vi "Autonomous Independent.vi"() -> ()   [LabVIEW 2014]
doc: "This VI is called when autonomous begins, and will automatically be terminated when autonomous ends. You can carry out timed or sensor driven robot movement independently without needing to return to the caller."
uses:
  <vilib>/Rock Robotics/WPI/Joystick/WPI_JoystickGetSetRefNum.vi
  Robot Global Data.vi
  <vilib>/Rock Robotics/WPI/RobotDrive/WPI_RobotDriveArcadeDrive_Standard(NoSaturation).vi
  <vilib>/Rock Robotics/WPI/SafetyOutput/WPI_SafetyOutputConfigMenu.ctl
  <vilib>/Rock Robotics/WPI/Relay/WPI_RelayValue.ctl
panel:
  out "Current Movement, for debugging":T1 {"Y Joystick Value" scale=1.0..-1.0; "X Joystick Value" scale=-1.0..1.0}
  in  "Array of robot movements":T2(array[cluster]) {"Y Joystick Value" scale=1.0..-1.0; "X Joystick Value" scale=-1.0..1.0}
  # "Be sure to right-click and choose Data Operations>>Make Current Value default if you want to save the array values with the VI"
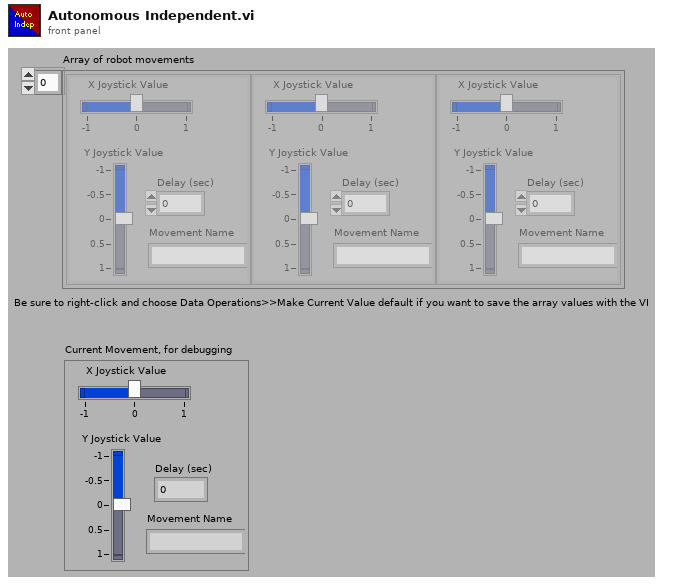
[diagram p1: front panel]
types:
  T1 = cluster{"X Joystick Value":dbl, "Y Joystick Value":dbl, "Delay (sec)":dbl, "Movement Name":string}
  T2 = cluster{"X Joystick Value":dbl, "Y Joystick Value":dbl, "Delay (sec)":dbl, "Movement Name":string}[]
  T3 = typedef "WPI_SafetyOutputConfigMenu.ctl" = enum16{"Enable", "Disable"}
  T4 = typedef "WPI_RelayValue.ctl" = enum16{"Off", "On", "Forward", "Reverse"}
  T5 = typedef "WPI_RobotDriveDevRef.ctl" = cluster{"DevStatus":errorcluster, "Motors[]":T6[], "Square Inputs":bool, "Max Output":dbl}
  T6 = typedef "WPI_MotorControlDeviceRef.ctl" = cluster{"DeviceStatus":errorcluster, "Type":enum16{"PWM", "CAN"}, "PWM":cluster{"Digital Module":T7, "PWM Channel":T8, "DeadBand":T9}, "CAN":cluster{"Device Number":u8, "Control Mode":T10, "Semaphore":T11, "Max Vout":dbl}, "Invert":bool, "TransformRef":T12, "InvTransformRef":T12}
  T7 = typedef "FPGA_TypedefDigitalModule.ctl" = enum16{"Digital Module 1", "Digital Module 2"}
  T8 = typedef "FPGA_DIOPWMChannel.ctl" = enum8{"PWM 1", "PWM 2", "PWM 3", "PWM 4", "PWM 5", "PWM 6", "PWM 7", "PWM 8", "PWM 9", "PWM 10", "Invalid"}
  T9 = typedef "WPI_PWMDeadband.ctl" = cluster{"Name":string, "maxPositivePwm":i32, "minPositivePwm":i32, "centerPwm":i32, "maxNegativePwm":i32, "minNegativePwm":i32, "angularRange":u16}
  T10 = typedef "WPI_CANJaguar_ControlMode.ctl" = enum8{"Percent VBus", "Current", "Speed", "Position", "Voltage"}
  T11 = typedef "Semaphore RefNum" = refnum<k1>
  T12 = typedef "WPI_PWMTransform_ConPane.ctl" = refnum<vi>
  T13 = typedef "WPI_GyroDevRef.ctl" = cluster{"DevStatus":errorcluster, "Analog Module":T14, "Analog Channel":T15, "Offset":dbl, "Gain (VoltsPerDegree/Second)":dbl}
  T14 = typedef "FPGA_TypedefAnalogModule.ctl" = enum16{"Analog Module 1", "Analog Module 2"}
  T15 = typedef "FPGA_AIChannel.ctl" = enum8{"AI 1", "AI 2", "AI 3", "AI 4", "AI 5", "AI 6", "AI 7", "AI 8", "Invalid"}
  T16 = typedef "WPI_RelayDevRef.ctl" = cluster{"DevStatus":errorcluster, "Relay Channel":T17, "Digital Module":T7, "Relay Direction":T18}
  T17 = typedef "FPGA_DIORelayChannel.ctl" = enum8{"Relay 1", "Relay 2", "Relay 3", "Relay 4", "Relay 5", "Relay 6", "Relay 7", "Relay 8", "Invalid"}
  T18 = typedef "WPI_RelayDirection.ctl" = enum16{"Both directions", "Forward only", "Reverse only"}
  T19 = typedef "WPI_JoystickDevRef.ctl" = cluster{"Device":T20}
  T20 = typedef "WPI_JoystickDeviceEnum.ctl" = enum16{"USB 0", "USB 1", "USB 2", "USB 3", "USB 4", "USB 5"}
  T21 = cluster{"axis 1 (x)":dbl, "axis 2 (y)":dbl, "axis 3 (throttle)":dbl, "axis 4":dbl, "axis 5":dbl, "axis 6":dbl}
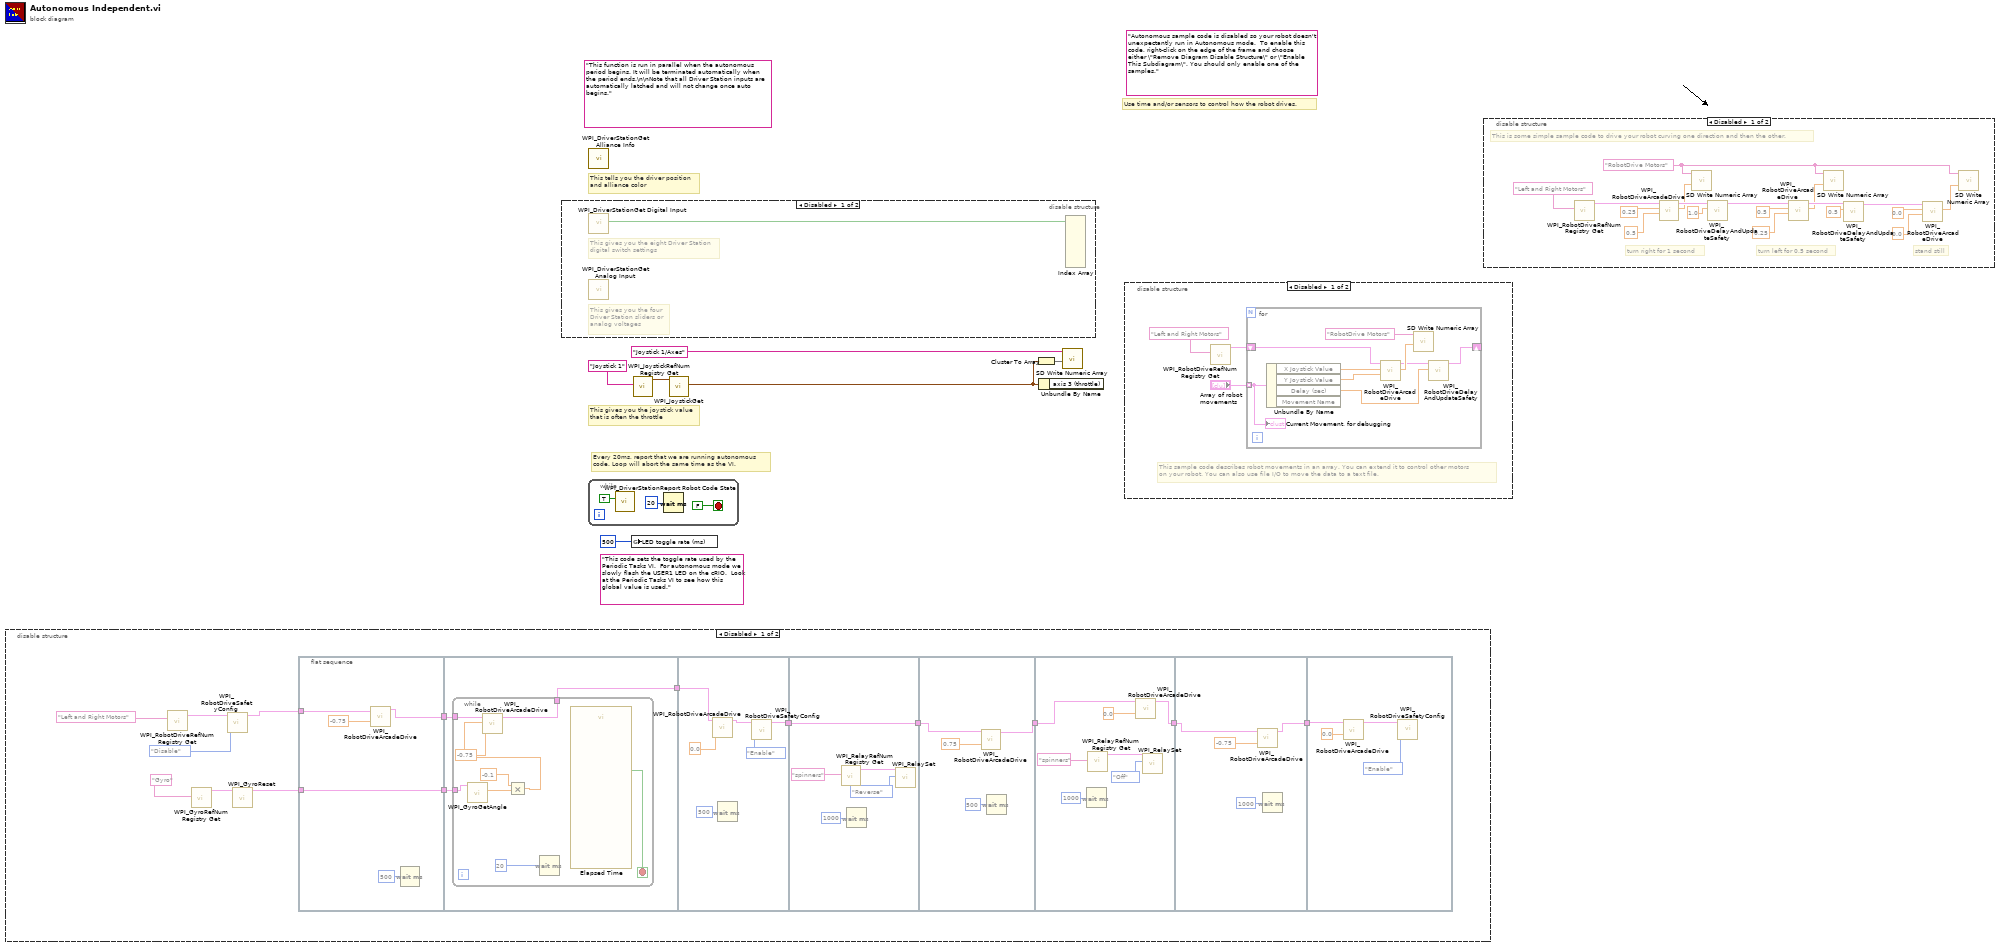
[diagram p0: block diagram]
diagram:
  (unwired) "This code sets the toggle rate used by the Periodic Tasks VI.  For autonomous mode we slowly flash the USER1 LED on the cRIO.  Look at the Periodic Tasks VI to see how this global value is used."
  (unwired) "Autonomous sample code is disabled so your robot doesn't unexpectantly run in Autonomous mode.  To enable this code, right-click on the edge of the frame and choose either \"Remove Diagram Disable Structure\" or \"Enable This Subdiagram\". You should only enable one of the samples."
  (unwired) "This function is run in parallel when the autonomous period begins. It will be terminated automatically when the period ends.\n\nNote that all Driver Station inputs are automatically latched and will not change once auto begins."
  # "Every 20ms, report that we are running autonomous\ncode. Loop will abort the same time as the VI."
  # "This gives you the joystick value\nthat is often the throttle"
  # "Use time and/or sensors to control how the robot drives."
  # "This tells you the driver position\nand alliance color"
  n1 = disable-structure shown="Disabled" {
    frame Disabled {
      n2 = call <vilib>:"WPI_RobotDriveRefNum Registry Get.vi"("refnum name"="Left and Right Motors") -> ("RobotDriveDevRef"=w12:T5)  [unwired: 9 in, 1 out]
      n3 = call <vilib>:"WPI_GyroRefNum Registry Get.vi"("refnum name"="Gyro") -> ("GyroDevRef"=w7:T13)  [unwired: 9 in, 1 out]
      n4 = call <vilib>:"WPI_RobotDriveSafetyConfig.vi"("mode"=WPI_SafetyOutputConfigMenu."Disable", "RobotDriveDevRef"=w12) -> ("RobotDriveDevRef"=w10:T5)  [unwired: 8 in, 1 out]
      n5 = call <vilib>:"WPI_GyroReset.vi"("GyroDevRef"=w7) -> ("GyroDevRef"=w9:T13)  [unwired: 9 in, 1 out]
      n6 = flat-sequence {
        tunnel: [w24] -> w21
        tunnel: w10 -> [w25]
        tunnel: w9 -> [w23]
        tunnel: [w23] -> w20
        tunnel: w21 -> [w27]
        tunnel: w20 -> [w28]
        tunnel: [w29] -> w19
        tunnel: [w40] -> w18
        tunnel: w19 -> [w41]
        tunnel: w18 -> [w49]
        tunnel: [w49] -> w17
        tunnel: w17 -> [w50]
        tunnel: [w51] -> w16
        tunnel: w16 -> [w58]
        tunnel: [w57] -> w15
        tunnel: w15 -> [w62]
        tunnel: [w61] -> w14
        tunnel: w14 -> [w65]
        frame #0 {
          n7 = call-poly <vilib>:"WPI_RobotDriveArcadeDrive.vi"("Y axis value"=-0.75, "RobotDriveDevRef"=w25) -> ("RobotDriveDevRef"=w24:T5)  [unwired: 7 in, 2 out]
          n8 = Wait (ms)(milliseconds to wait=u32 500) -> ()  [unwired: 1 out]
        }
        frame #1 {
          n9 = while {
            tunnel: [w31] -> w29
            tunnel: w28 -> [w36]
            tunnel: w27 -> [w32]
            stop <- w38 stop-if-true
            n10 = call <vilib>:"WPI_GyroGetAngle.vi"("GyroDevRef"=w36) -> ("Angle"=w34:dbl)  [unwired: 7 in, 3 out]
            n11 = Multiply(x=-0.1, y=w34) -> (x*y=w33:dbl)
            n12 = call-poly <vilib>:"WPI_RobotDriveArcadeDrive.vi"("Y axis value"=-0.75, "X axis value"=w33, "RobotDriveDevRef"=w32) -> ("RobotDriveDevRef"=w31:T5)  [unwired: 6 in, 2 out]
            n13 = Wait (ms)(milliseconds to wait=u32 20) -> ()  [unwired: 1 out]
            n14 = call "Elapsed Time"() -> ("Time has Elapsed"=w38:bool)  [unwired: 12 in, 7 out]
          }
        }
        frame #2 {
          n15 = call-poly <vilib>:"WPI_RobotDriveArcadeDrive.vi"("Y axis value"=0.0, "RobotDriveDevRef"=w41) -> ("RobotDriveDevRef"=w43:T5)  [unwired: 7 in, 2 out]
          n16 = Wait (ms)(milliseconds to wait=u32 500) -> ()  [unwired: 1 out]
          n17 = call <vilib>:"WPI_RobotDriveSafetyConfig.vi"("mode"=WPI_SafetyOutputConfigMenu."Enable", "RobotDriveDevRef"=w43) -> ("RobotDriveDevRef"=w40:T5)  [unwired: 8 in, 1 out]
        }
        frame #3 {
          n18 = call <vilib>:"WPI_RelayRefNum Registry Get.vi"("refnum name"="spinners") -> ("RelayDevRef"=w46:T16)  [unwired: 9 in, 1 out]
          n19 = Wait (ms)(milliseconds to wait=u32 1000) -> ()  [unwired: 1 out]
          n20 = call <vilib>:"WPI_RelaySet.vi"("RelayValue"=WPI_RelayValue."Reverse", "RelayDevRef"=w46) -> ()  [unwired: 8 in, 2 out]
        }
        frame #4 {
          n21 = call-poly <vilib>:"WPI_RobotDriveArcadeDrive.vi"("Y axis value"=0.75, "RobotDriveDevRef"=w50) -> ("RobotDriveDevRef"=w51:T5)  [unwired: 7 in, 2 out]
          n22 = Wait (ms)(milliseconds to wait=u32 500) -> ()  [unwired: 1 out]
        }
        frame #5 {
          n23 = Wait (ms)(milliseconds to wait=u32 1000) -> ()  [unwired: 1 out]
          n24 = call <vilib>:"WPI_RelayRefNum Registry Get.vi"("refnum name"="spinners") -> ("RelayDevRef"=w56:T16)  [unwired: 9 in, 1 out]
          n25 = call-poly <vilib>:"WPI_RobotDriveArcadeDrive.vi"("Y axis value"=0.0, "RobotDriveDevRef"=w58) -> ("RobotDriveDevRef"=w57:T5)  [unwired: 7 in, 2 out]
          n26 = call <vilib>:"WPI_RelaySet.vi"("RelayValue"=WPI_RelayValue."Off", "RelayDevRef"=w56) -> ()  [unwired: 8 in, 2 out]
        }
        frame #6 {
          n27 = call-poly <vilib>:"WPI_RobotDriveArcadeDrive.vi"("Y axis value"=-0.75, "RobotDriveDevRef"=w62) -> ("RobotDriveDevRef"=w61:T5)  [unwired: 7 in, 2 out]
          n28 = Wait (ms)(milliseconds to wait=u32 1000) -> ()  [unwired: 1 out]
        }
        frame #7 {
          n29 = call-poly <vilib>:"WPI_RobotDriveArcadeDrive.vi"("Y axis value"=0.0, "RobotDriveDevRef"=w65) -> ("RobotDriveDevRef"=w67:T5)  [unwired: 7 in, 2 out]
          n30 = call <vilib>:"WPI_RobotDriveSafetyConfig.vi"("mode"=WPI_SafetyOutputConfigMenu."Enable", "RobotDriveDevRef"=w67) -> ()  [unwired: 8 in, 2 out]
        }
      }
    }
    frame Enabled {
    }
  }
  n31 = disable-structure shown="Disabled" {
    frame Disabled {
      # "This gives you the eight Driver Station\ndigital switch settings"
      # "This gives you the four\nDriver Station sliders or\nanalog voltages"
      n32 = call <vilib>:"WPI_DriverStationGet Digital Input.vi"() -> ("Driver Station Digital Input (1-8)"=w69:bool[])  [unwired: 11 out]
      n33 = call <vilib>:"WPI_DriverStationGet Analog Input.vi"() -> ()  [unwired: 12 out]
      n34 = Index Array(array=w69) -> ()  [unwired: 8 in, 8 out]
    }
    frame Enabled {
    }
  }
  n35 = while {
    stop <- FALSE stop-if-true
    n36 = call <vilib>:"WPI_DriverStationReport Robot Code State.vi"("Autonomous"=TRUE) -> ()  [unwired: 10 in, 1 out]
    n37 = Wait (ms)(milliseconds to wait=u32 20) -> ()  [unwired: 1 out]
  }
  n38 = call <vilib>:"WPI_DriverStationGet Alliance Info.vi"() -> ()  [unwired: 12 out]
  n39 = global write "Robot Global Data.vi" "LED toggle rate (ms)"(u32 500 ("LED ms toggle rate")) -> ()
  n40 = call <vilib>:"WPI_JoystickRefNum Registry Get.vi"("refnum name"="Joystick 1") -> ("JoystickDevRef"=w5:T19)  [unwired: 1 in, 9 out]
  n41 = call <vilib>:"WPI_JoystickGet.vi"("JoystickDevRef"=w5) -> ("Axes"=w2:T21)  [unwired: 1 in, 5 out]
  n42 = Cluster To Array(cluster=w2) -> (array=w3:dbl[])
  n43 = Unbundle By Name(w2) -> ()  [unwired: 1 out]
  n44 = call <vilib>:"SD Write Numeric Array.vi"("Numeric Array"=w3, "Name"="Joystick 1/Axes") -> ()  [unwired: 8 in, 2 out]
  n45 = disable-structure shown="Disabled" {
    frame Disabled {
      # "This sample code describes robot movements in an array. You can extend it to control other motors\non your robot. You can also use file I/O to move the data to a text file."
      n46 = call <vilib>:"WPI_RobotDriveRefNum Registry Get.vi"("refnum name"="Left and Right Motors") -> ("RobotDriveDevRef"=w74:T5)  [unwired: 1 in, 9 out]
      n47 = for {
        shift-right: [w80] -> _
        shift-left: w74 -> [w81]
        tunnel: "Array of robot movements" -> [w76] mode=indexing
        n48 = Unbundle By Name(w76) -> ("X Joystick Value"=w79:dbl, "Y Joystick Value"=w78:dbl, "Delay (sec)"=w77:dbl)  [unwired: 1 out]
        n49 = call-poly <vilib>:"WPI_RobotDriveArcadeDrive.vi"("Y axis value"=w78, "X axis value"=w79, "RobotDriveDevRef"=w81) -> ("Motor Values"=w83:dbl[], "RobotDriveDevRef"=w82:T5)  [unwired: 1 in, 6 out]
        n50 = call <vilib>:"SD Write Numeric Array.vi"("Numeric Array"=w83, "Name"="RobotDrive Motors") -> ()  [unwired: 8 in, 2 out]
        n51 = call <vilib>:"WPI_RobotDriveDelayAndUpdateSafety.vi"("Delay (s)"=w77, "RobotDriveDevRef"=w82) -> ("RobotDriveDevRef 2"=w80:T5)  [unwired: 8 in, 1 out]
        "Current Movement, for debugging" <- w76
      }
    }
    frame Enabled {
    }
  }
  n52 = disable-structure shown="Disabled" {
    frame Disabled {
      w85 = "RobotDrive Motors" ("Name")
      # "This is some simple sample code to drive your robot curving one direction and then the other."
      # "stand still"
      # "turn left for 0.5 second"
      # "turn right for 1 second"
      n53 = call <vilib>:"WPI_RobotDriveRefNum Registry Get.vi"("refnum name"="Left and Right Motors") -> ("RobotDriveDevRef"=w89:T5)  [unwired: 1 in, 9 out]
      n54 = call-poly <vilib>:"WPI_RobotDriveArcadeDrive.vi"("Y axis value"=0.5 ("X axis value"), "X axis value"=0.25, "RobotDriveDevRef"=w89) -> ("Motor Values"=w88:dbl[], "RobotDriveDevRef"=w96:T5)  [unwired: 1 in, 6 out]
      n55 = call <vilib>:"SD Write Numeric Array.vi"("Numeric Array"=w88, "Name"=w85) -> ()  [unwired: 8 in, 2 out]
      n56 = call <vilib>:"WPI_RobotDriveDelayAndUpdateSafety.vi"("Delay (s)"=1.0, "RobotDriveDevRef"=w96) -> ("RobotDriveDevRef 2"=w95:T5)  [unwired: 8 in, 1 out]
      n57 = call-poly <vilib>:"WPI_RobotDriveArcadeDrive.vi"("Y axis value"=0.25 ("X axis value"), "X axis value"=0.5, "RobotDriveDevRef"=w95) -> ("Motor Values"=w87:dbl[], "RobotDriveDevRef"=w94:T5)  [unwired: 1 in, 6 out]
      n58 = call <vilib>:"SD Write Numeric Array.vi"("Numeric Array"=w87, "Name"=w85) -> ()  [unwired: 8 in, 2 out]
      n59 = call <vilib>:"WPI_RobotDriveDelayAndUpdateSafety.vi"("Delay (s)"=0.5, "RobotDriveDevRef"=w94) -> ("RobotDriveDevRef 2"=w93:T5)  [unwired: 8 in, 1 out]
      n60 = call-poly <vilib>:"WPI_RobotDriveArcadeDrive.vi"("Y axis value"=0.0 ("X axis value"), "X axis value"=0.0, "RobotDriveDevRef"=w93) -> ("Motor Values"=w86:dbl[])  [unwired: 1 in, 7 out]
      n61 = call <vilib>:"SD Write Numeric Array.vi"("Numeric Array"=w86, "Name"=w85) -> ()  [unwired: 8 in, 2 out]
    }
    frame Enabled {
    }
  }
